vi "GETSubData.vi"(10 "Variable Header":string, 11 "Data out":string[][](array[string])) -> (3 "delimiter (Tab)":string)   [LabVIEW 2011]
panel:
  out "shot NR":string
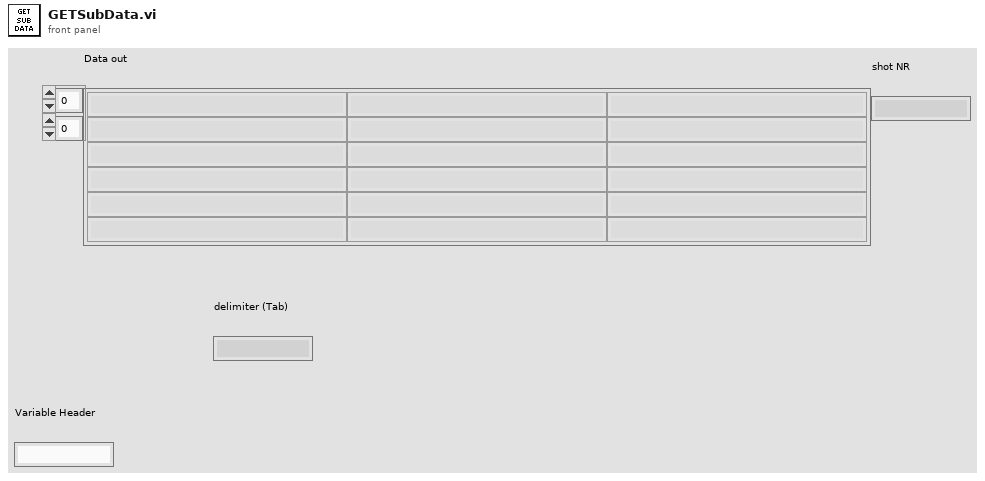
[diagram p1: front panel]
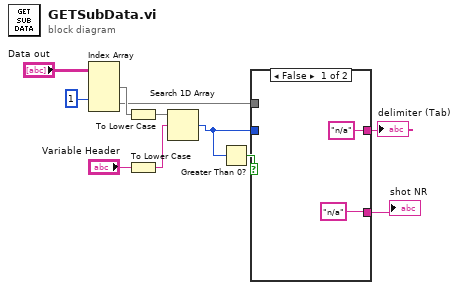
[diagram p0: block diagram]
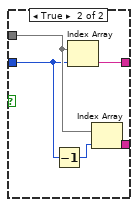
[diagram p2: hidden frame]
diagram:
  n1 = Index Array(array="Data out", index (row) #2=1 ("index (row)")) -> (element #1=w8:string[], element #2=w4:string[])  [unwired: 3 in]
  n2 = To Lower Case(string=w8) -> (all lower case string=w7:string[])
  n3 = To Lower Case(string="Variable Header") -> (all lower case string=w5:string)
  n4 = Search 1D Array(1D array=w7, element=w5) -> (index of element=w2:i32)  [unwired: 1 in]
  n5 = Greater Than 0?(x=w2) -> (x > 0?=w1:bool)
  n6 = case shown="False" w1 {
    tunnel: ["n/a" ("delimiter (Tab)") w18] -> w10
    tunnel: w4 -> [_ w17]
    tunnel: ["n/a" ("delimiter (Tab)") w15] -> w3
    tunnel: w2 -> [_ w14]
    frame False {
    }
    frame True {
      n7 = Decrement(x=w14) -> (x-1=w16:i32)
      n8 = Index Array(array=w17, index=w14) -> (element=w18:string)
      n9 = Index Array(array=w17, index=w16) -> (element=w15:string)
    }
  }
  "delimiter (Tab)" <- w10
  "shot NR" <- w3
